vi "Get Class Members.vi"(8 "error in (no error)":errorcluster, 11 "Class Name":string) -> (0 "error out":errorcluster, 1 "Success?":bool, 3 "Member Map":T1)   [LabVIEW 2020, in "ClassLoader.lvlib"]
doc: "Return a map containing all the members for the given class.\n\nThis VI does not automatically load data. Front-load before calling this VI!"
uses:
  ClassLoader.lvlib
  Sub/Ctl/Ctl_Member Map.ctl
  <vilib>/Utility/Data Type/Member VI Info.ctl
  Sub/Cache/Cache_Members Global.vi
  <vilib>/Utility/config.llb/NI_LVConfig.lvlib
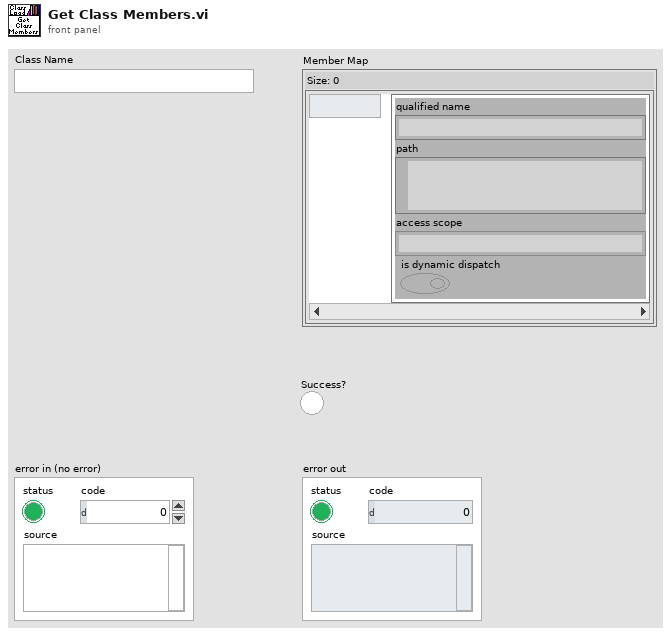
[diagram p1: front panel]
types:
  T1 = typedef "ClassLoader.lvlib/Ctl_Member Map.ctl" = map{string, T2}
  T2 = typedef "Member VI Info.ctl" = cluster{"qualified name":string, "path":path, "access scope":enum32{"invalid scope", "public", "private", "protected", "community"}, "is dynamic dispatch":bool}
  T3 = typedef "NI_LVConfig.lvlib/Config Data RefNum.ctl" = refnum<k1>
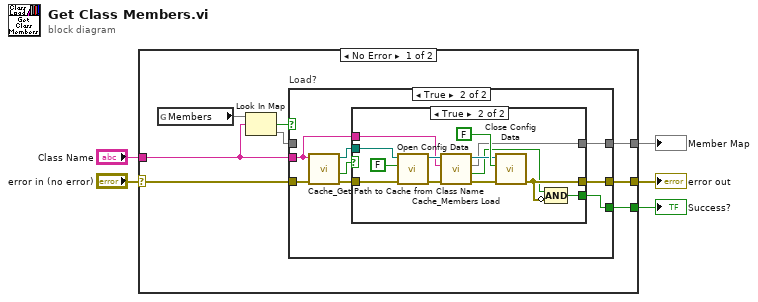
[diagram p0: block diagram]
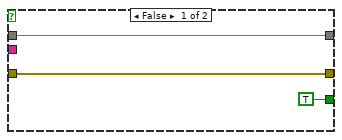
[diagram p2: hidden frame]
diagram:
  n1 = case shown="No Error" "error in (no error)" {
    selector: "error in (no error)" -> [w13 w39]
    tunnel: "Class Name" -> [w9 _]
    tunnel: [w12 w39] -> w3
    tunnel: [w11 _] -> w2
    tunnel: [w10 _] -> w1
    frame No Error {
      n2 = global read "Cache_Members Global.vi" "Members"() -> (w6:map{string, T1})
      n3 = Look In Map(map=w6, key=w9) -> (key not found?=w8:bool, value=w7:T1)  [unwired: 1 in]
      n4 = case "Load?" shown="True" w8 {
        tunnel: w13 -> [w15 w24]
        tunnel: [w15 w20] -> w12
        tunnel: [TRUE w19] -> w11
        tunnel: [w16 w18] -> w10
        tunnel: w9 -> [_ w17]
        tunnel: w7 -> [w16 _]
        frame False {
        }
        frame True {
          n5 = call "Cache_Get Path to Cache from Class Name.vi"("error in (no error)"=w24, "Class Name"=w17) -> ("error out"=w21:errorcluster, "Success?"=w22:bool, "Cache Path"=w23:path)  [unwired: 7 in]
          n6 = case shown="True" w22 {
            tunnel: w23 -> [_ w36]
            tunnel: w17 -> [_ w28]
            tunnel: w21 -> [w25 w35]
            tunnel: [w25 w34] -> w20
            tunnel: [_ w33] -> w19
            tunnel: [_ w30] -> w18
            frame False {
            }
            frame True {
              n7 = call <vilib>:"Open Config Data.vi"("error in (no error)"=w35, "create file if necessary (T)"=FALSE, "configuration file path"=w36) -> ("error out"=w27:errorcluster, "refnum"=w32:T3)  [unwired: 6 in, 1 out]
              n8 = call "Cache_Members Load.vi"("error in (no error)"=w27, "Class Name"=w28, "Refnum in"=w32) -> ("error out"=w26:errorcluster, "Success?"=w29:bool, "Member Map"=w30:T1, "Refnum out"=w31:T3)  [unwired: 5 in]
              n9 = call <vilib>:"Close Config Data.vi"("error in (no error)"=w26, "write file if changed (T)"=FALSE, "refnum"=w31) -> ("error out"=w34:errorcluster)  [unwired: 7 in, 1 out]
              n10 = Compound Arithmetic op=AND(w29, invert w34) -> (w33:bool)
            }
          }
        }
      }
    }
    frame Error {
    }
  }
  "error out" <- w3
  "Success?" <- w2
  "Member Map" <- w1
